vi "eTdsBLE_Test_WithEvent.vi"() -> ()   [LabVIEW 2013]
uses:
  D:/GitHub/GT-Bionics/TDS-HM/Labview Code/C# BLE Interface/eTDS BLE Interface/TdsBleInterface for LV/TdsForLV/TdsForLV/bin/TdsForLV.dll
  TdsForLV/TdsForLV/bin/TdsForLV.dll
panel:
  out "DeviceName":string
  in  "stop":bool
  out "BleDataArray":u8[](array[numeric])
  out "error out":errorcluster
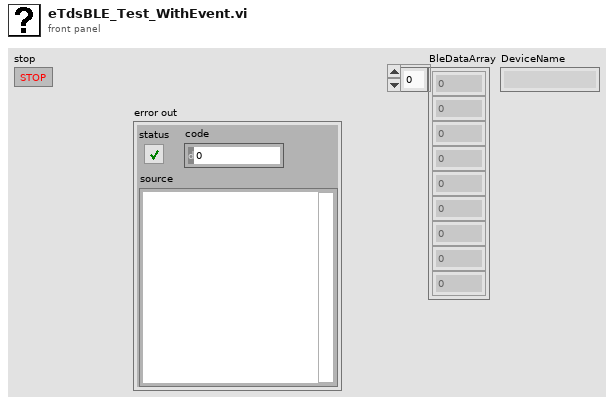
[diagram p1: front panel]
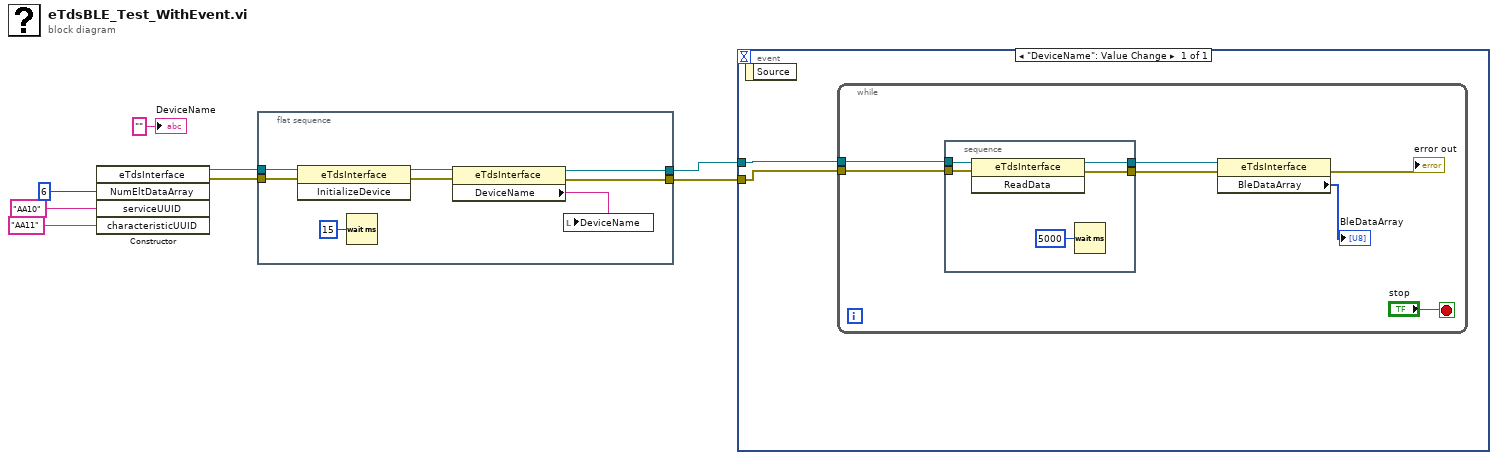
[diagram p0: block diagram]
diagram:
  n1 = constructor class="eTdsInterface"("NumEltDataArray"=6, "serviceUUID"="AA10", "characteristicUUID"="AA11") -> (reference out=w8:refnum<k24>, error out=w7:errorcluster)  [unwired: 3 in, 4 out]
  n2 = flat-sequence {
    tunnel: w8 -> [w16]
    tunnel: w7 -> [w15]
    tunnel: [w11] -> w3
    tunnel: [w10] -> w2
    frame #0 {
      n3 = invoke class="eTdsInterface" method="InitializeDevice"(reference=w16, error in=w15) -> (reference out=w13:refnum<k24>, error out=w12:errorcluster)  [unwired: 1 in, 1 out]
      n4 = Wait (ms)(milliseconds to wait=u32 15) -> ()  [unwired: 1 out]
      n5 = property class="eTdsInterface"(reference=w13, error in=w12) -> (reference out=w11:refnum<k24>, error out=w10:errorcluster, "DeviceName"=w9:string)
      n6 = local write "DeviceName"(w9) -> ()
    }
  }
  n7 = event shown="[0] \"DeviceName\": Value Change" {
    selector: _ -> [_]
    dyn-events: _ -> [_]
    timeout: _ -> [_]
    tunnel: w3 -> [w18]
    tunnel: w2 -> [w17]
    event "DeviceName": Value Change {
      n8 = event-data() -> ()  [unwired: 1 in, 1 out]
      n9 = while {
        tunnel: w18 -> [w25]
        tunnel: w17 -> [w19]
        stop <- "stop" stop-if-true
        n10 = stacked-sequence {
          tunnel: w25 -> [w30]
          tunnel: w19 -> [w29]
          tunnel: [w28] -> w22
          tunnel: [w27] -> w21
          frame #0 {
            n11 = invoke class="eTdsInterface" method="ReadData"(reference=w30, error in=w29) -> (reference out=w28:refnum<k24>, error out=w27:errorcluster)  [unwired: 1 in, 1 out]
            n12 = Wait (ms)(milliseconds to wait=u32 5000) -> ()  [unwired: 1 out]
          }
        }
        n13 = property class="eTdsInterface"(reference=w22, error in=w21) -> (error out=→"error out":errorcluster, "BleDataArray"=→"BleDataArray":u8[])  [unwired: 1 out]
      }
    }
  }
  "DeviceName" <- "" ("DeviceName")
